vi "GDSError_ReportError.vi"(5 "error in (no error)":errorcluster) -> (19 "error out":errorcluster)   [LabVIEW 2012]
doc: "You can use this VI to generate errors."
uses:
  <resource>/Framework/Providers/Open_GDS/ClassProviders/Common/Error/private/GDSError_LogCases.ctl
  <vilib>/Utility/error.llb/DialogType.ctl
  <resource>/Framework/Providers/Open_GDS/SubVIs/GOOP_ErrorCodes.ctl
panel:
  in  "Close":bool
  out "Error String":string
  # "A system error has occurred"
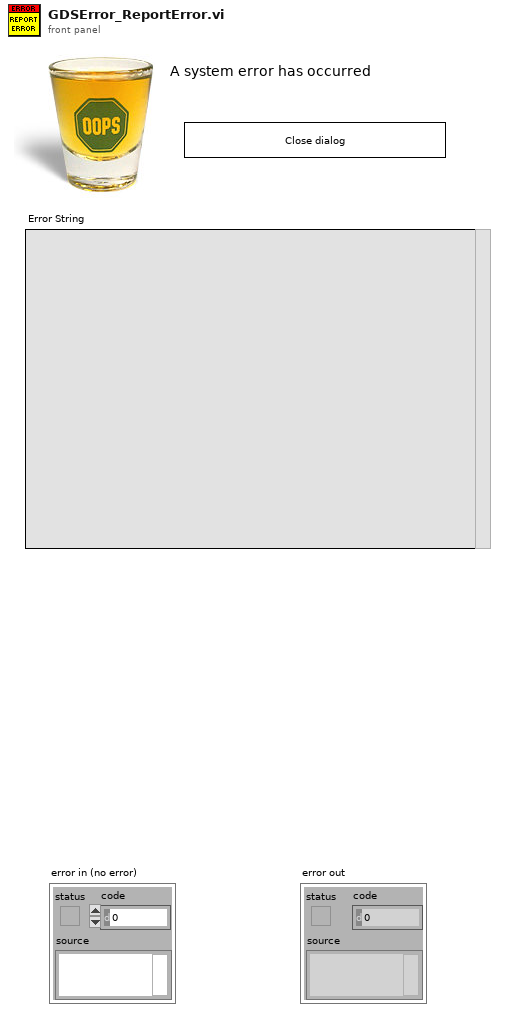
[diagram p1: front panel]
types:
  T1 = typedef "GDSError_LogCases.ctl" = enum16{"Init", "AddError", "ReadFirstError", "ReadLatestError", "ReadAllErrors", "ClearError", "ClearAllErrors"}
  T2 = enum32{"None", "Stop", "Question", "Exclamation", "Information"}
  T3 = cluster{"Counter":i32, "Text":string, "Email":string}
  T4 = enum16{"open", "replace", "create", "open or create", "replace or create", "replace or create with confirmation"}
  T5 = typedef "GOOP_ErrorCodes.ctl" = enum16{"LicenseFileMissing", "LicenseFileNotCorrect", "NoProductAccessGranted", "AgreementNoAccepted", "NoValidProviderFound", "LicenseExpired", "LanguageUndefined", "LanguageFileMissing", "LanguageFileChecksumError", "DublicateLanguageTranslation", "LanguageStringIDNotFound", "CommunityLimitReached", "ClassFileLocked", "ClassFileReadOnly", "ProjectNotValid"}
  T6 = typedef "DialogType.ctl" = u16
  T7 = typedef "LVRectTypeDef.ctl" = cluster{"Left":i16, "Top":i16, "Right":i16, "Bottom":i16}
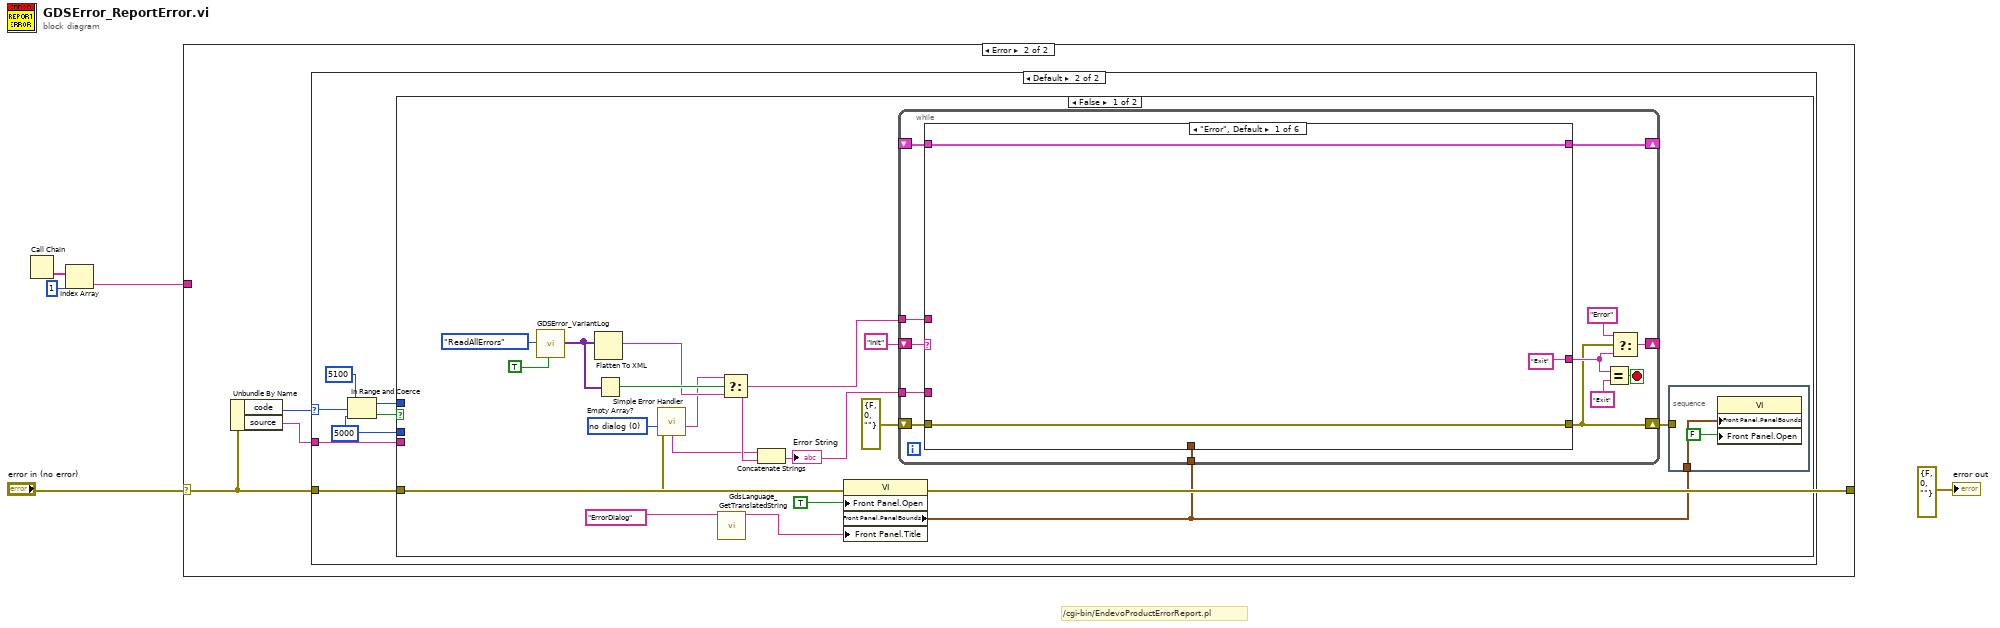
[diagram p0: block diagram]
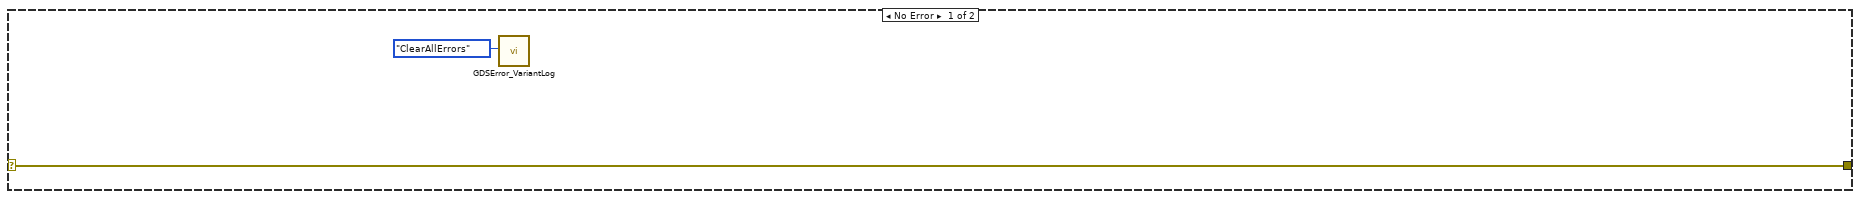
[diagram p2: hidden frame]
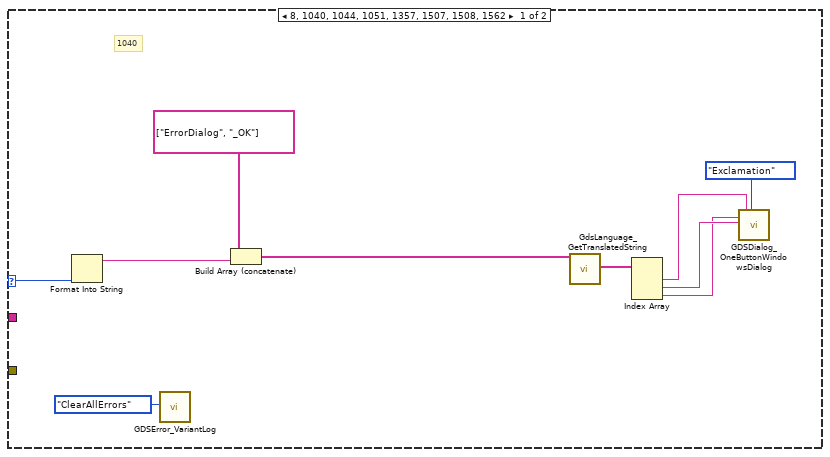
[diagram p3: hidden frame]
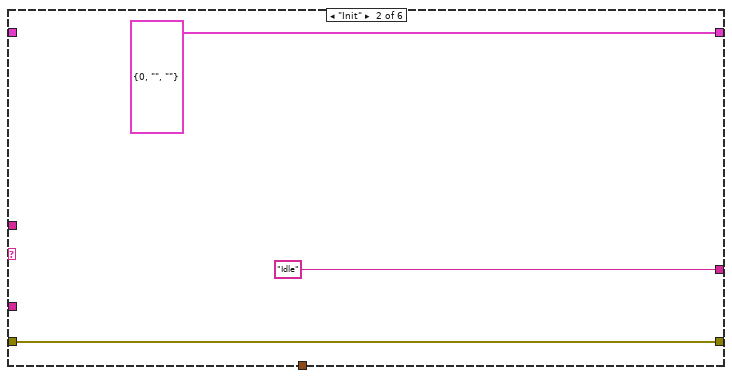
[diagram p4: hidden frame]
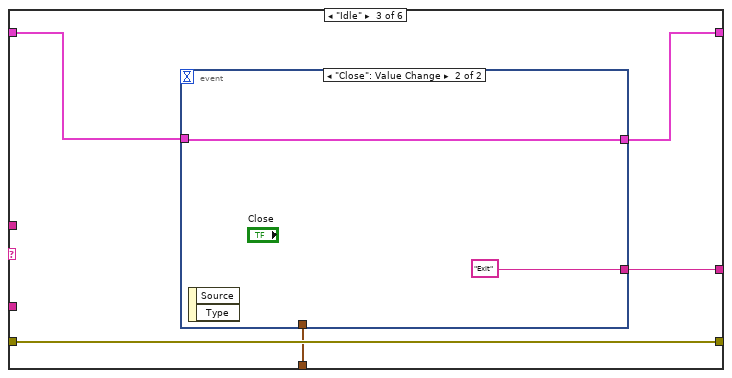
[diagram p5: hidden frame]
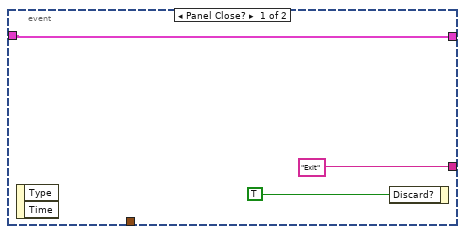
[diagram p6: hidden frame]
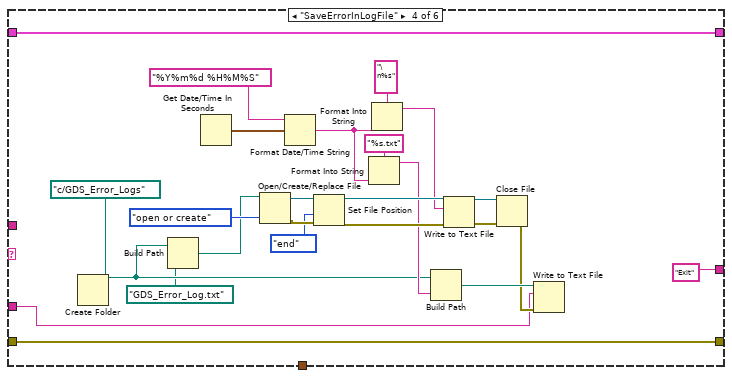
[diagram p7: hidden frame]
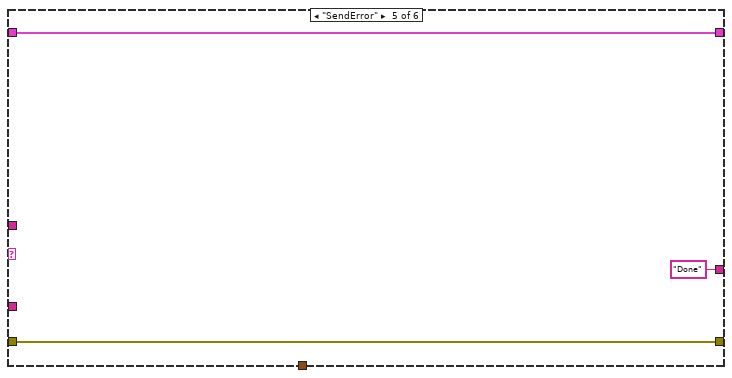
[diagram p8: hidden frame]
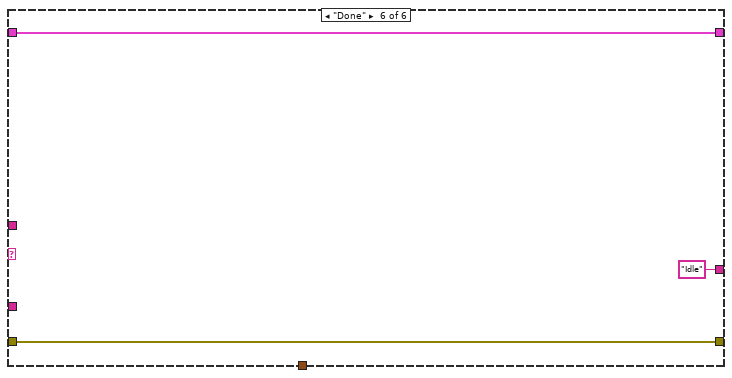
[diagram p9: hidden frame]
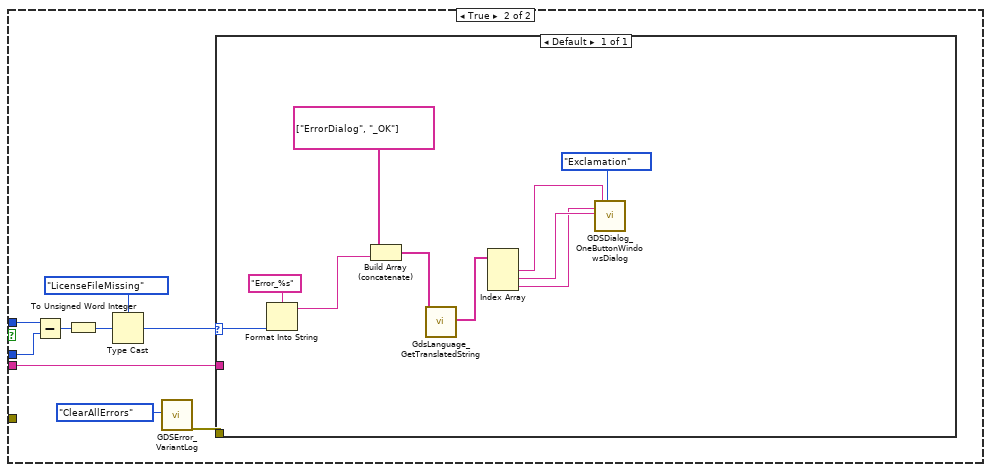
[diagram p10: hidden frame]
diagram:
  # "/cgi-bin/EndevoProductErrorReport.pl"
  n1 = Call Chain() -> (call chain=w4:string[])
  n2 = Index Array(array=w4, index=1) -> (element=w2:string)
  n3 = case shown="Error" "error in (no error)" {
    selector: "error in (no error)" -> [w7 w10]
    tunnel: [w7 w10] -> _
    tunnel: w2 -> [_ _]
    frame No Error {
      n4 = call <resource>:"GDSError_VariantLog.vi"("cases"=GDSError_LogCases."ClearAllErrors") -> ()  [unwired: 17 in, 2 out]
    }
    frame Error {
      n5 = Unbundle By Name(w10) -> ("code"=w9:i32, "source"=w8:string)
      n6 = case shown="Default" w9 {
        selector: w9 -> [w11 w22]
        tunnel: w10 -> [_ w27]
        tunnel: w8 -> [_ w21]
        frame 8, 1040, 1044, 1051, 1357, 1507, 1508, 1562 {
          # "1040"
          n7 = Format Into String(w11) -> (resulting string=w18:string)  [unwired: 3 in, 1 out]
          n8 = call <resource>:"GDSError_VariantLog.vi"("cases"=GDSError_LogCases."ClearAllErrors") -> ()  [unwired: 17 in, 2 out]
          n9 = Build Array (concatenate)(string[] ["ErrorDialog", "_OK"], w18) -> (w17:string[])
          n10 = call <resource>:"GdsLanguage_GetTranslatedString.vi"("StringID(s)"=w17) -> ("StringsOut"=w16:string[])  [unwired: 15 in, 3 out]
          n11 = Index Array(array=w16) -> (element #1=w15:string, element #2=w14:string, element #3=w13:string)  [unwired: 3 in]
          n12 = call <resource>:"GDSDialog_OneButtonWindowsDialog.vi"("UserText"=w13, "ButtonName"=w14, "DialogTitle"=w15, "Icon"=T2."Exclamation") -> ()  [unwired: 13 in, 3 out]
        }
        frame Default {
          w23 = 5000 ("y")
          n13 = In Range and Coerce(upper limit=5100, x=w22, lower limit=w23) -> (coerced(x)=w24:i32, In Range?=w25:bool)
          n14 = case shown="False" w25 {
            tunnel: w27 -> [w34 _]
            tunnel: w24 -> [_ w116]
            tunnel: w23 -> [_ w115]
            tunnel: w21 -> [_ w109]
            frame False {
              w42 = T6 0 items=["no dialog", "OK message", "continue or stop message", "OK message + warnings", "continue/stop + warnings"] ("type of dialog (OK msg:1)")
              n15 = call <resource>:"GDSError_VariantLog.vi"("cases"=GDSError_LogCases."ReadAllErrors", "DeleteWhenRead"=TRUE) -> ("ErrorArray"=w40:variant[])  [unwired: 16 in, 1 out]
              n16 = Flatten To XML(anything=w40) -> (xml string=w39:string)
              n17 = Empty Array?(array=w40) -> (empty?=w41:bool)
              n18 = call <vilib>:"Simple Error Handler.vi"("type of dialog (OK msg:1)"=w42, "error in (no error)"=w34) -> ("source out"=w33:string, "message"=w31:string)  [unwired: 3 in, 3 out]
              n19 = call <resource>:"GdsLanguage_GetTranslatedString.vi"("StringID(s)"="ErrorDialog") -> ("FirstStringOut"=w29:string)  [unwired: 15 in, 3 out]
              n20 = Select(t=w33, s=w41, f=w39) -> (s? t:f=w32:string)
              n21 = Concatenate Strings(w31, w32) -> (w28:string)
              "Error String" <- w28
              n22 = property class="VI"("Front Panel.Open"=TRUE ("Front Panel Window:Open"), "Front Panel.Title"=w29) -> ("Front Panel.PanelBounds"=w35:T7)  [unwired: 2 in, 2 out]
              n23 = while {
                shift-right: [w53] -> w36
                shift-left: errorcluster {"status"=FALSE, "code"=0, "source"=""} ("error IO") -> [w60]
                shift-right: [w58] -> _
                shift-left: "Init" -> [w59]
                shift-right: [w52] -> _
                shift-left: _ -> [w51]
                tunnel: w35 -> [w50]
                tunnel: w32 -> [w49]
                tunnel: w28 -> [w48]
                stop <- w57 stop-if-true
                n24 = case shown="\"Error\", Default" w59 {
                  tunnel: w60 -> [w63 w65 w70 w99 w103 w105]
                  tunnel: [w63 w65 w70 w99 w103 w105] -> w53
                  tunnel: ["Exit" "Idle" w71 "Exit" "Done" "Idle"] -> w54
                  tunnel: [w61 T3 {"Counter"=0, "Text"="", "Email"=""} w67 w101 w102 w107] -> w52
                  tunnel: w51 -> [w61 _ w68 w101 w102 w107]
                  tunnel: w50 -> [_ _ w69 _ _ _]
                  tunnel: w49 -> [_ _ _ _ _ _]
                  tunnel: w48 -> [_ _ _ w77 _ _]
                  frame "Error", Default {
                  }
                  frame "Init" {
                  }
                  frame "Idle" {
                    n25 = event shown="[1] \"Close\": Value Change" {
                      selector: _ -> [_ _]
                      dyn-events: _ -> [_ _]
                      timeout: _ -> [_ _]
                      tunnel: ["Exit" "Exit"] -> w71
                      tunnel: w69 -> [_ _]
                      tunnel: w68 -> [w72 w75]
                      tunnel: [w72 w75] -> w67
                      event Panel Close? {
                        n26 = event-data() -> ()  [unwired: 1 in, 2 out]
                        n27 = event-data("Discard?"=TRUE) -> ()  [unwired: 1 in, 1 out]
                      }
                      event "Close": Value Change {
                        n28 = event-data() -> ()  [unwired: 1 in, 2 out]
                      }
                    }
                  }
                  frame "SaveErrorInLogFile" {
                    n29 = Create Folder(path (use dialog)=path "c:/GDS_Error_Logs" ("file path (use dialog)")) -> (created path=w80:path)  [unwired: 2 in, 2 out]
                    n30 = Build Path(base path=w80, name or relative path=path "GDS_Error_Log.txt" ("file path (use dialog)")) -> (appended path=w78:path)
                    n31 = Get Date/Time In Seconds() -> (seconds since 1Jan1904=w92:timestamp)
                    n32 = Open/Create/Replace File(file path (use dialog)=w78, operation (0:open)=T4."open or create") -> (refnum out=w98:refnum<file>, error out=w97:errorcluster)  [unwired: 4 in, 1 out]
                    n33 = Format Date/Time String(time format string (%c)="%Y%m%d %H%M%S", seconds (now)=w92) -> (date/time string=w86:string)  [unwired: 1 in]
                    n34 = Set File Position(refnum=w98, from (0:start)=enum16{"start", "end", "current"}."end", error in=w97) -> (refnum out=w95:refnum<file>, error out=w94:errorcluster)  [unwired: 1 in]
                    n35 = Format Into String(format string="%s.txt", w86) -> (resulting string=w84:string)  [unwired: 2 in, 1 out]
                    n36 = Format Into String(format string="\n%s", w86) -> (resulting string=w89:string)  [unwired: 2 in, 1 out]
                    n37 = Build Path(base path=w80, name or relative path=w84) -> (appended path=w83:path)
                    n38 = Write to Text File(file (use dialog)=w95, text=w89, error in=w94) -> (refnum out=w87:refnum<file>, error out=w88:errorcluster)  [unwired: 1 in, 1 out]
                    n39 = Close File(refnum=w87, error in=w88) -> (error out=w82:errorcluster)  [unwired: 1 out]
                    n40 = Write to Text File(file (use dialog)=w83, text=w77, error in=w82) -> ()  [unwired: 1 in, 3 out]
                  }
                  frame "SendError" {
                  }
                  frame "Done" {
                  }
                }
                n41 = Equal?(x=w54, y="Exit") -> (x = y?=w57:bool)
                n42 = Select(t="Error", s=w53, f=w54) -> (s? t:f=w58:string)
              }
              n43 = stacked-sequence {
                tunnel: w36 -> [_]
                tunnel: w35 -> [w47]
                frame #0 {
                  n44 = property class="VI"("Front Panel.PanelBounds"=w47, "Front Panel.Open"=FALSE ("Front Panel Window:Open")) -> ()  [unwired: 2 in, 2 out]
                }
              }
            }
            frame True {
              n45 = Subtract(x=w116, y=w115) -> (x-y=w114:i32)
              n46 = To Unsigned Word Integer(number=w114) -> (unsigned 16bit integer=w113:u16)
              n47 = Type Cast(type=GOOP_ErrorCodes."LicenseFileMissing" ("UserDefinedCodes(+5000)"), x=w113) -> (*(type *) &x=w111:T5)
              n48 = call <resource>:"GDSError_VariantLog.vi"("cases"=GDSError_LogCases."ClearAllErrors") -> ("error out"=w108:errorcluster)  [unwired: 17 in, 1 out]
              n49 = case shown="Default" w111 {
                selector: w111 -> [w117]
                tunnel: w109 -> [_]
                tunnel: w108 -> [_]
                frame Default {
                  n50 = Format Into String(format string="Error_%s", w117) -> (resulting string=w123:string)  [unwired: 2 in, 1 out]
                  n51 = Build Array (concatenate)(string[] ["ErrorDialog", "_OK"], w123) -> (w122:string[])
                  n52 = call <resource>:"GdsLanguage_GetTranslatedString.vi"("StringID(s)"=w122) -> ("StringsOut"=w121:string[])  [unwired: 15 in, 3 out]
                  n53 = Index Array(array=w121) -> (element #1=w120:string, element #2=w119:string, element #3=w118:string)  [unwired: 3 in]
                  n54 = call <resource>:"GDSDialog_OneButtonWindowsDialog.vi"("UserText"=w118, "ButtonName"=w119, "DialogTitle"=w120, "Icon"=T2."Exclamation") -> ()  [unwired: 13 in, 3 out]
                }
              }
            }
          }
        }
      }
    }
  }
  "error out" <- errorcluster {"status"=FALSE, "code"=0, "source"=""} ("error IO")
